vi "Sanity check arb plane entry.vi"(10 "ROI Setup":T1[](array[typedef]) {"Z stop" format="%#_6f"; "Z start" format="%#_6f"; "ROI group ID" format="%#_6f"; "Laser Power (%)" format="%#_6f"; "Zoom" format="%#_6f"; "Frame Size" format="%#_6f"; "Number of lines" format="%#_6f"; "Composite ID" format="%#_6f"; "Angle (deg)" format="%#_6f"; "ROI Time (ns)" format="%#_6f"; "ROI ID" format="%#_6f"; "Pixels in ROI" format="%#_6f"; "ROI index" format="%#_6f"; "Y stop" format="%#_6f"; "X stop" format="%#_6f"; "X start" format="%#_6f"; "Y start" format="%#_6f"}, 11 "ROI management Input cluster":T2) -> (3 "Prevent new POI":bool)   [LabVIEW 2017]
uses:
  Typedefs/ROI management Input cluster.ctl
  Typedefs/ROI ID Enum.ctl
  Visualisation/Functional Imaging Viewer/Typedefs/ROI parameters data type.ctl
  ROI Entry screen/Globals/gl_ROI Entry UI globals.vi
panel:
  # "X Start\nY Start\nX Stop\nY Stop"
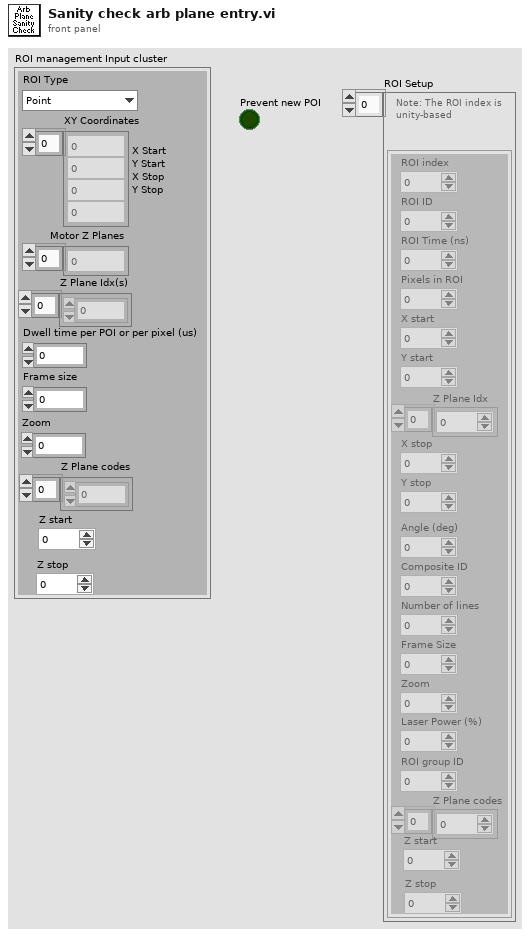
[diagram p1: front panel]
types:
  T1 = typedef "ROI parameters data type.ctl" = cluster{"ROI index":dbl, "ROI ID":dbl, "ROI Time (ns)":dbl, "Pixels in ROI":dbl, "X start":dbl, "Y start":dbl, "X stop":dbl, "Y stop":dbl, "Angle (deg)":dbl, "Composite ID":dbl, "Number of lines":dbl, "Frame Size":dbl, "Zoom":dbl, "Laser Power (%)":dbl, "ROI group ID":dbl, "Z Plane Idx":i32[], "Z Plane codes":u8[], "Z start":dbl, "Z stop":dbl}
  T2 = typedef "ROI management Input cluster.ctl" = cluster{"ROI Type":T3, "XY Coordinates":i32[], "Motor Z Planes":dbl[], "Dwell time per POI or per pixel (us)":dbl, "Frame size":i32, "Zoom":dbl, "Z Plane Idx(s)":i32[], "Z Plane codes":u8[], "Z start":dbl, "Z stop":dbl}
  T3 = typedef "ROI ID Enum.ctl" = enum16{"Point", "MiniScan", "Comp. MiniScan", "Rectangle", "Comp. volume", "Arb. plane point"}
  T4 = typedef "ROI entry screen ctrl refs cluster.ctl" = cluster{"Done button":refnum<vi>, "Imaging button":refnum<vi>, "Acquisition button":refnum<vi>, "POI dwell time (us)":refnum<vi>, "Scan dwell time per pixel (us)":refnum<vi>, "# of planes":refnum<vi>, "Zoom Ctrl":refnum<vi>, "Equal size":refnum<vi>, "Channel":refnum<vi>, "Image Display":refnum<vi>, "Z-Plane Selector":refnum<vi>, "Number of lines left":refnum<vi>, "Z-stack folder path":refnum<vi>, "POI Density":refnum<vi>, "Arb Plane Entry":refnum<vi>, "Whole plane":refnum<vi>, "Clear Last":refnum<vi>, "Clear All":refnum<vi>, "Trial Length (sec)":refnum<vi>, "Palette Type":refnum<vi>, "Intensity slider":refnum<vi>, "# POI":refnum<vi>, "Max Z Proj":refnum<vi>, "Zplane ind":refnum<vi>, "Wavelength (nm)":refnum<vi>, "Number of Trials":refnum<vi>, "Funct stim.trig.enable":refnum<vi>, "Funct stim.trig.delay (s)":refnum<vi>, "Line Mode":refnum<vi>, "Step size (µm)":refnum<vi>, "ROI move mode":refnum<vi>, "Cool-down time (s)":refnum<vi>, "Enable cool-down time":refnum<vi>, "Motor Z ind. (um)":refnum<vi>, "AOL Z ind. (um)":refnum<vi>, "Load Reference Image":refnum<vi>}
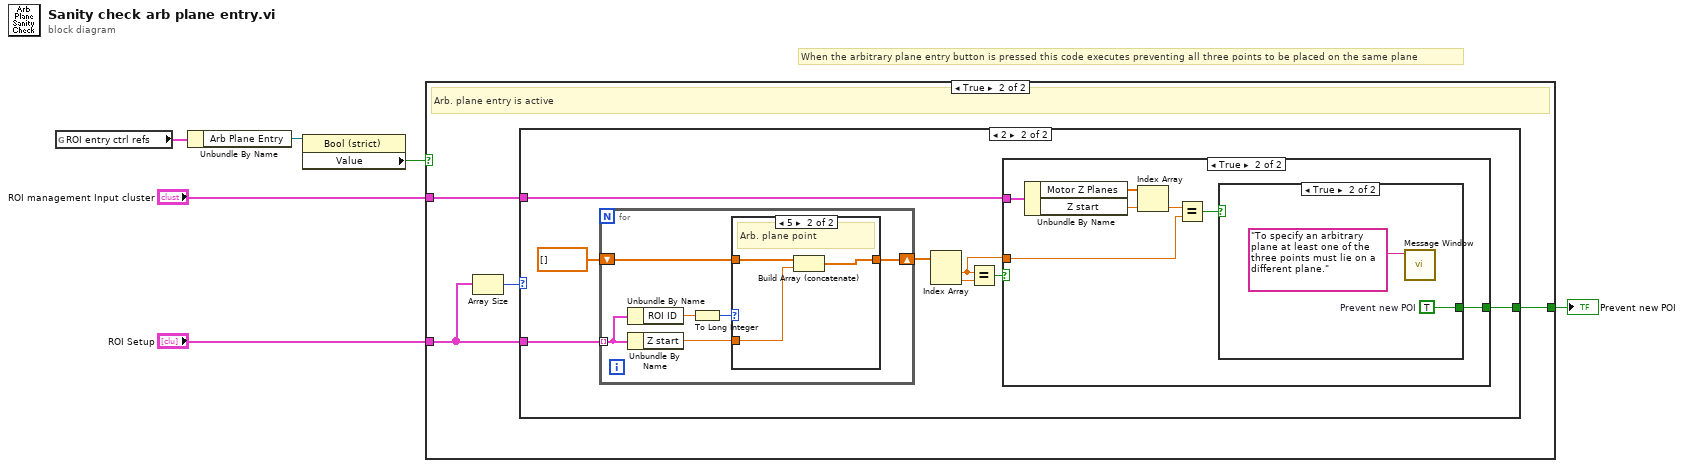
[diagram p0: block diagram]
diagram:
  # "When the arbitrary plane entry button is pressed this code executes preventing all three points to be placed on the same plane"
  n1 = global read "gl_ROI Entry UI globals.vi" "ROI entry ctrl refs"() -> (w2:T4)
  n2 = Unbundle By Name(w2) -> ("Arb Plane Entry"=w3:refnum<vi>)
  n3 = property class="Bool (strict)"(reference=w3) -> ("Value"=w1:bool)  [unwired: 1 in, 2 out]
  n4 = case shown="True" w1 {
    tunnel: [_ w10] -> w6
    tunnel: "ROI management Input cluster" -> [_ w9]
    tunnel: "ROI Setup" -> [_ w8]
    frame False {
      # "Arb. plane entry is not active"
    }
    frame True {
      # "Arb. plane entry is active"
      n5 = Array Size(array=w8) -> (size(s)=w7:i32)
      n6 = case shown="2" w7 {
        tunnel: w8 -> [_ w16]
        tunnel: w9 -> [_ w15]
        tunnel: [_ w12] -> w10
        frame Default {
        }
        frame 2 {
          n7 = for {
            tunnel: w16 -> [w33] mode=indexing
            shift-right: [w30] -> w18
            shift-left: dbl[] [] ("appended array") -> [w29]
            n8 = Unbundle By Name(w33) -> ("ROI ID"=w32:dbl)
            n9 = Unbundle By Name(w33) -> ("Z start"=w28:dbl)
            n10 = To Long Integer(number=w32) -> (32bit integer=w31:i32)
            n11 = case shown="5" w31 {
              tunnel: [w34 w37] -> w30
              tunnel: w29 -> [w34 w36]
              tunnel: w28 -> [_ w35]
              frame Default {
              }
              frame 5 {
                # "Arb. plane point"
                n12 = Build Array (concatenate)(w36, w35) -> (w37:dbl[])
              }
            }
          }
          n13 = Index Array(array=w18) -> (element #1=w13:dbl, element #2=w17:dbl)  [unwired: 2 in]
          n14 = Equal?(x=w13, y=w17) -> (x = y?=w14:bool)
          n15 = case shown="True" w14 {
            tunnel: w15 -> [_ w25]
            tunnel: w13 -> [_ w21]
            tunnel: [_ w19] -> w12
            frame False {
            }
            frame True {
              n16 = Unbundle By Name(w25) -> ("Motor Z Planes"=w24:dbl[], "Z start"=w23:dbl)
              n17 = Index Array(array=w24, index=w23) -> (element=w22:dbl)
              n18 = Equal?(x=w22, y=w21) -> (x = y?=w20:bool)
              n19 = case shown="True" w20 {
                tunnel: [_ w26] -> w19
                frame False {
                }
                frame True {
                  w26 = TRUE  # Prevent new POI
                  n20 = call "Message Window.vi"("Message string"="To specify an arbitrary plane at least one of the three points must lie on a different plane.") -> ()  [unwired: 10 in, 1 out]
                }
              }
            }
          }
        }
      }
    }
  }
  "Prevent new POI" <- w6
